vi "IVI_save.vi"(4 "ext format":string=".ch_a#", 7 "Seq":string, 8 "error in":errorcluster, 9 "Waveform Data":waveform(dbl)[](graph)=[{"t0"=timestamp(-4.999999999588667e-07 s since 1904-01-01), "dt"=5e-10, "Y"=array[2000 elements]}, {"t0"=timestamp(-4.999999999588667e-07 s since 1904-01-01), "dt"=5e-10, "Y"=array[2000 elements]}], 10 "Channels":T2[](array[typedef])=[{"channel name"="CHANNEL1", "probe attenuation"=1.0, "vertical offset"=0.0, "vertical range"=10.0, "vertical coupling (DC)"=1, "save format"="%.6f"}, {"channel name"="CHANNEL1", "probe attenuation"=1.0, "vertical offset"=0.0, "vertical range"=10.0, "vertical coupling (DC)"=1, "save format"="%.6f"}] {"vertical coupling (DC)" items=["AC", "DC", "GND"]; "vertical range" format="%.3f"; "vertical offset" format="%.3f"; "probe attenuation" format="%.3f"}, 11 "Data Save":path[](array[path])) -> (0 "error out":errorcluster, 3 "dup Data Save":path[](array[path]))   [LabVIEW 2013]
uses:
  Acquisition/IVI_chan.ctl
  <vilib>/Utility/file.llb/Write To Spreadsheet File (DBL).vi
panel:
  in  "Json_template":T1
  out "JSON string":string
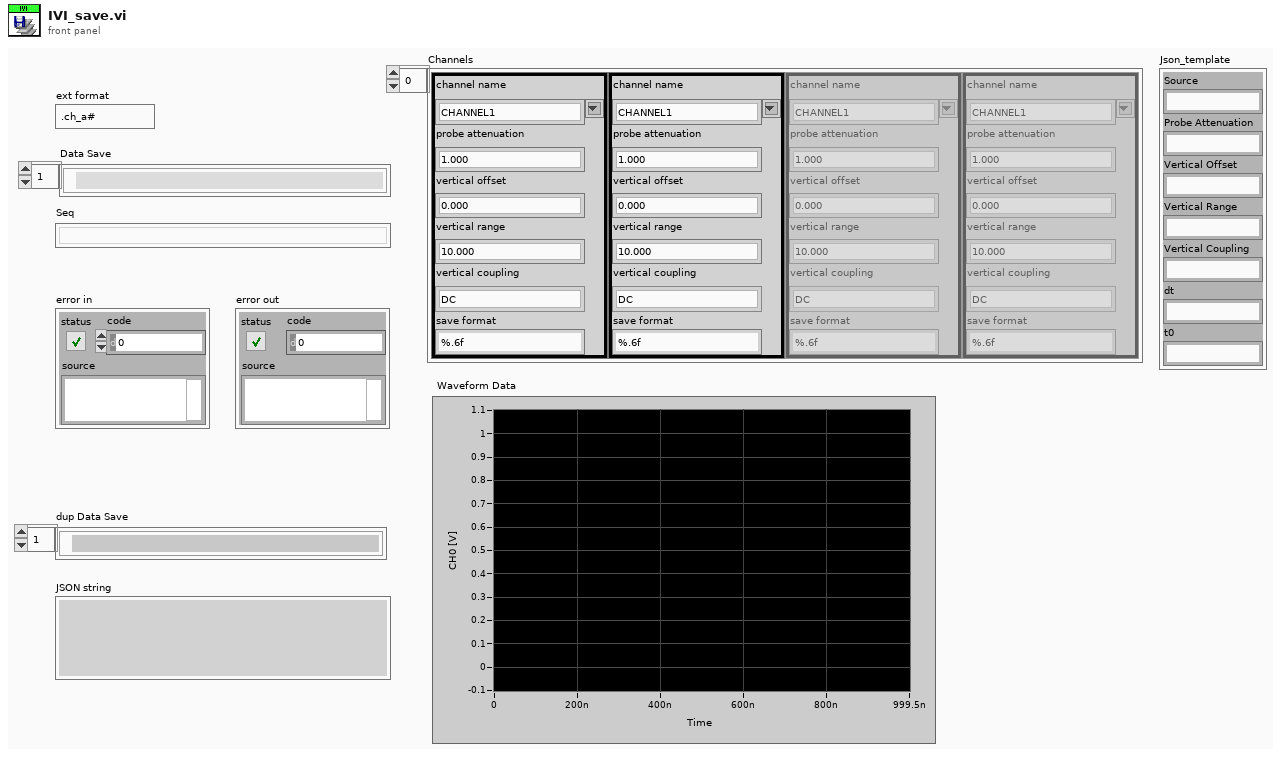
[diagram p1: front panel]
types:
  T1 = cluster{"Source":string, "Probe Attenuation":string, "Vertical Offset":string, "Vertical Range":string, "Vertical Coupling":string, "dt":string, "t0":string}
  T2 = typedef "IVI_chan.ctl" = cluster{"channel name":string, "probe attenuation":dbl, "vertical offset":dbl, "vertical range":dbl, "vertical coupling (DC)":i32, "save format":string}
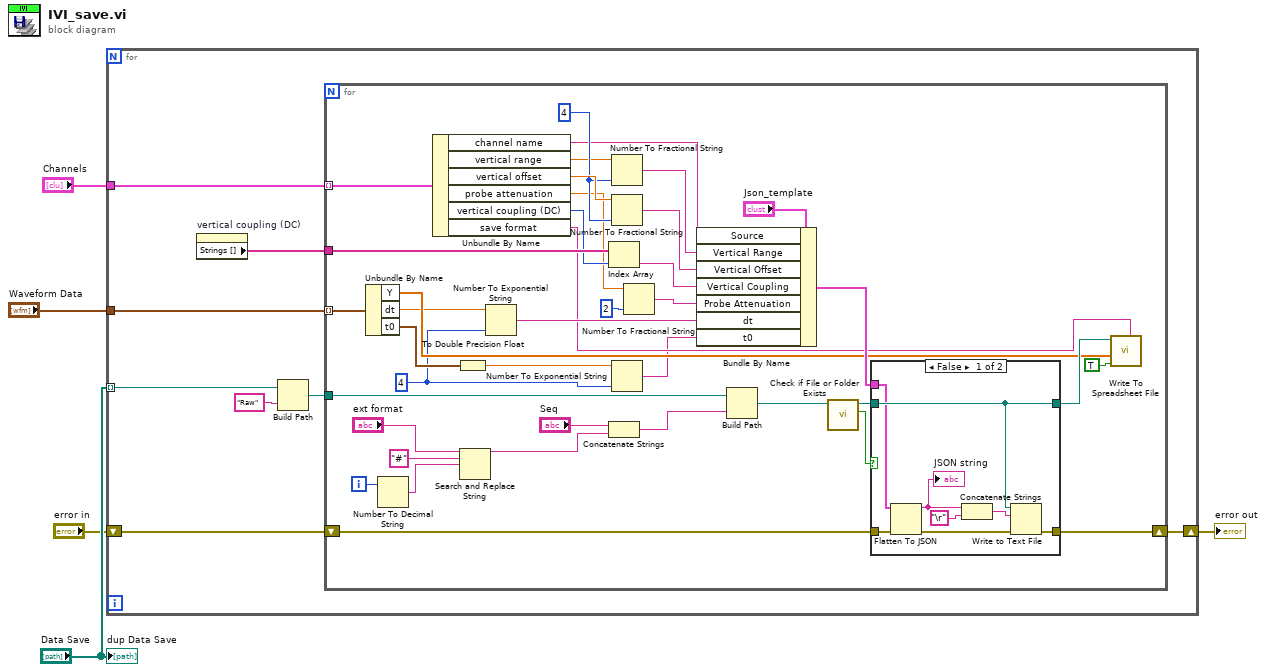
[diagram p0: block diagram]
diagram:
  n1 = for {
    tunnel: "Data Save" -> [w9] mode=indexing
    shift-right: [w12] -> w3
    shift-left: "error in" -> [w13]
    tunnel: "Channels" -> [w8]
    tunnel: "Waveform Data" -> [w7]
    n2 = property on="vertical coupling (DC)" class="Ring (strict)"() -> ("Strings []"=w6:string[])  [unwired: 2 in, 2 out]
    n3 = Build Path(base path=w9, name or relative path="Raw") -> (appended path=w11:path)
    n4 = for {
      tunnel: w11 -> [w52]
      tunnel: w8 -> [w45] mode=indexing
      tunnel: w7 -> [w24] mode=indexing
      shift-right: [w47] -> w12
      shift-left: w13 -> [w46]
      tunnel: w6 -> [w38]
      i -> [w29]
      w34 = i16 4 ("precision (6)")
      w18 = i16 4 ("precision (6)")
      n5 = Unbundle By Name(w24) -> ("Y"=w23:dbl[], "dt"=w21:dbl, "t0"=w20:timestamp)
      n6 = Number To Decimal String(number=w29) -> (decimal integer string=w30:string)  [unwired: 1 in]
      n7 = Unbundle By Name(w45) -> ("channel name"=w16:string, "vertical range"=w33:dbl, "vertical offset"=w36:dbl, "probe attenuation"=w14:dbl, "vertical coupling (DC)"=w15:i32, "save format"=w22:string)
      n8 = To Double Precision Float(number=w20) -> (double precision float=w19:dbl)
      n9 = Search and Replace String(input string="ext format", search string="#", replace string=w30) -> (result string=w26:string)  [unwired: 5 in, 3 out]
      n10 = Number To Exponential String(number=w21, precision (6)=w18) -> (E-format string=w41:string)  [unwired: 2 in]
      n11 = Index Array(array=w38, index=w15) -> (element=w37:string)
      n12 = Concatenate Strings("Seq", w26) -> (w25:string)
      n13 = Number To Fractional String(number=w33, precision (6)=w34) -> (F-format string=w32:string)  [unwired: 2 in]
      n14 = Number To Fractional String(number=w36, precision (6)=w34) -> (F-format string=w35:string)  [unwired: 2 in]
      n15 = Number To Exponential String(number=w19, precision (6)=w18) -> (E-format string=w17:string)  [unwired: 2 in]
      n16 = Number To Fractional String(number=w14, precision (6)=i16 2) -> (F-format string=w39:string)  [unwired: 2 in]
      n17 = Bundle By Name(cluster="Json_template", "Source"=w16, "Vertical Range"=w32, "Vertical Offset"=w35, "Vertical Coupling"=w37, "Probe Attenuation"=w39, "dt"=w41, "t0"=w17) -> (w43:T1)
      n18 = Build Path(base path=w52, name or relative path=w25) -> (appended path=w51:path)
      n19 = call <vilib>:"Check if File or Folder Exists.vi"("path"=w51) -> ("file or folder exists?"=w50:bool, "dup path"=w49:path)  [unwired: 8 in, 1 out]
      n20 = case shown="False" w50 {
        tunnel: w49 -> [w60 w62]
        tunnel: [w60 w62] -> w48
        tunnel: [w59 w61] -> w47
        tunnel: w46 -> [w57 w61]
        tunnel: w43 -> [w56 _]
        frame False {
          n21 = Flatten To JSON(anything=w56, error in (no error)=w57) -> (JSON string=w55:string, 11:w58:errorcluster)  [unwired: 1 in]
          "JSON string" <- w55
          n22 = Concatenate Strings(w55, "\r") -> (w53:string)
          n23 = Write to Text File(file (use dialog)=w60, text=w53, error in=w58) -> (error out=w59:errorcluster)  [unwired: 1 in, 2 out]
        }
        frame True {
        }
      }
      n24 = call-poly <vilib>:"Write To Spreadsheet File.vi"("format (%.3f)"=w22, "append to file? (new file:F)"=TRUE, "1D data"=w23, "file path (dialog if empty)"=w48) -> ()  [unwired: 4 in, 1 out]
    }
  }
  "error out" <- w3
  "dup Data Save" <- "Data Save"
